vi "Create RPC Method.vi"(8 "error in (no error)":errorcluster, 10 "RPC Method Parameters":T1, 11 "Server class in":refnum<vi>) -> (0 "error out":errorcluster, 2 "Newly created ?":bool, 3 "Server class out":refnum<vi>)   [LabVIEW 2019, in "gRPC Scripting Tools.lvlib"]
uses:
  gRPC Scripting Tools.lvlib
  TypeDefs/RPC Method Parameters.ctl
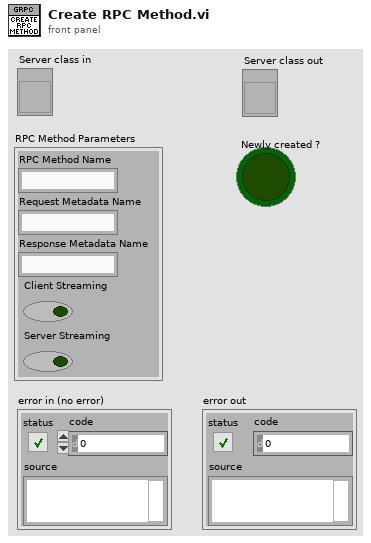
[diagram p1: front panel]
types:
  T1 = typedef "gRPC Scripting Tools.lvlib/RPC Method Parameters.ctl" = cluster{"RPC Method Name":string, "Request Metadata Name":string, "Response Metadata Name":string, "Client Streaming":bool, "Server Streaming":bool}
  T2 = enum32{"invalid VI type", "Standard VI", "Control VI", "Global VI", "Polymorphic VI", "Configuration VI", "SubSystem", "Facade VI", "Method VI"}
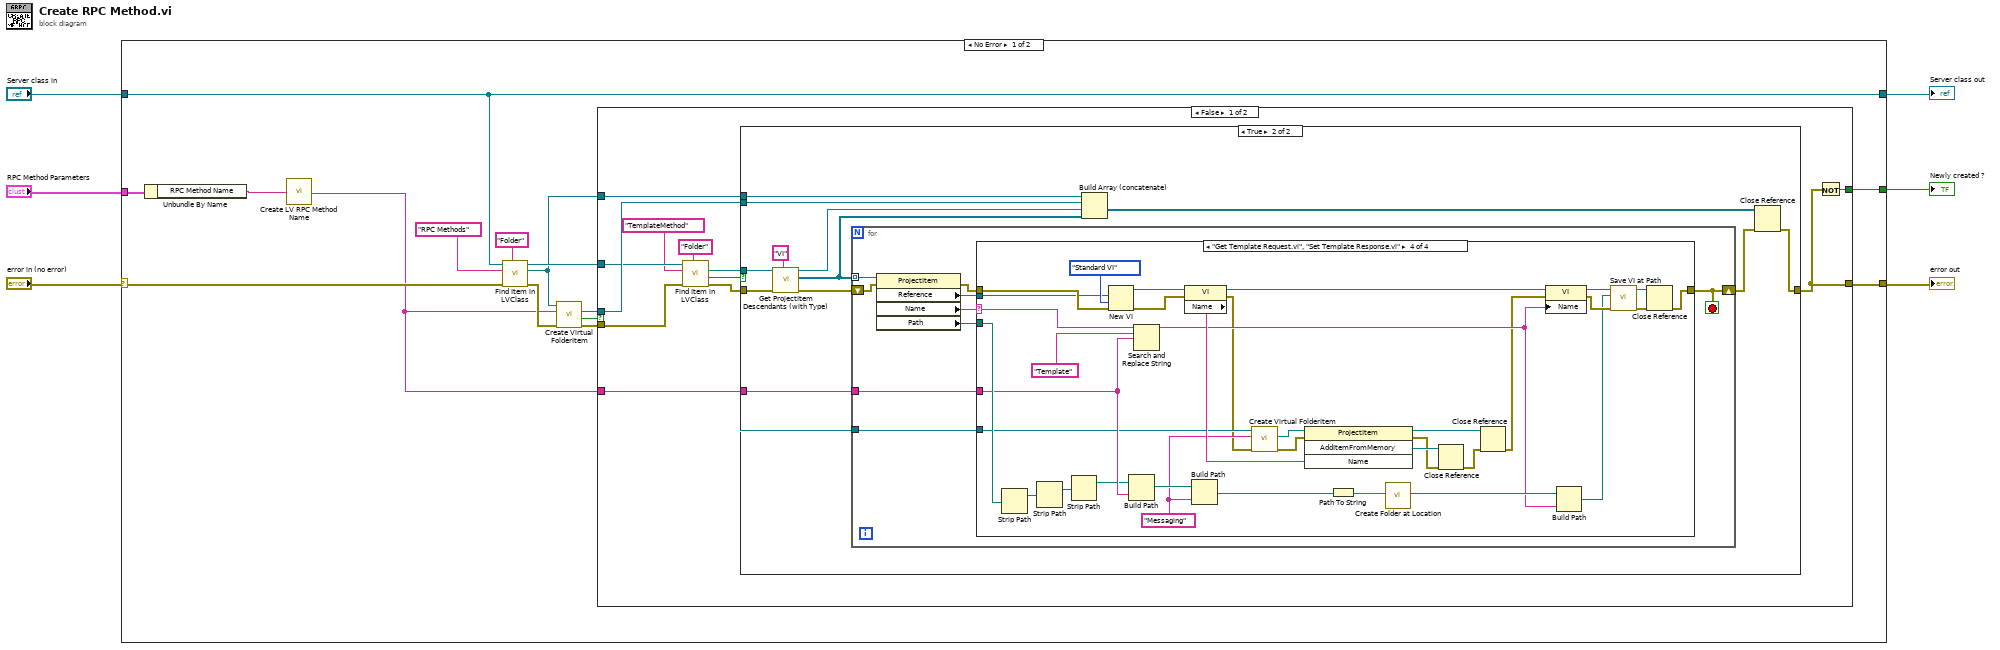
[diagram p0: block diagram]
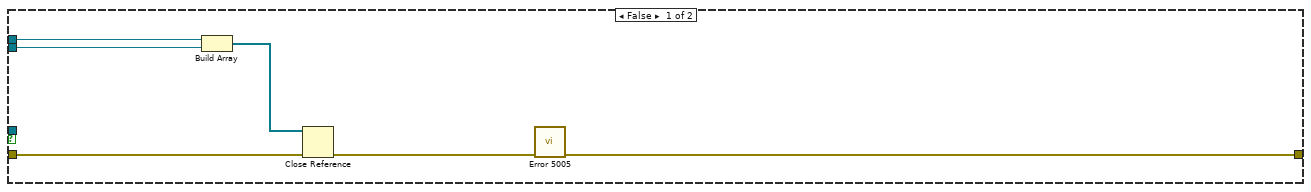
[diagram p2: hidden frame]
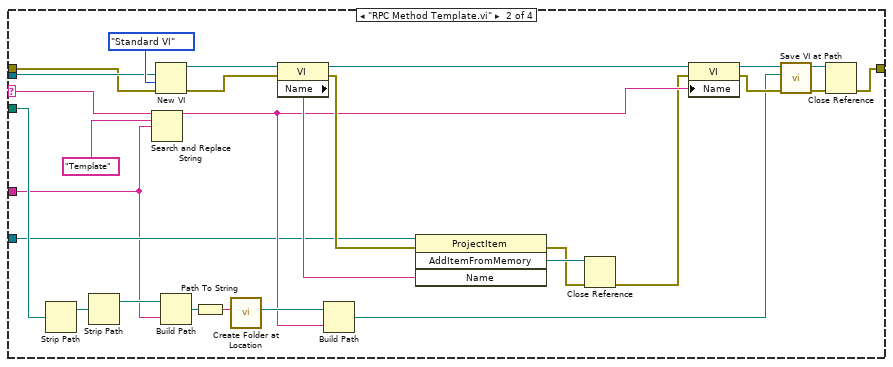
[diagram p4: hidden frame]
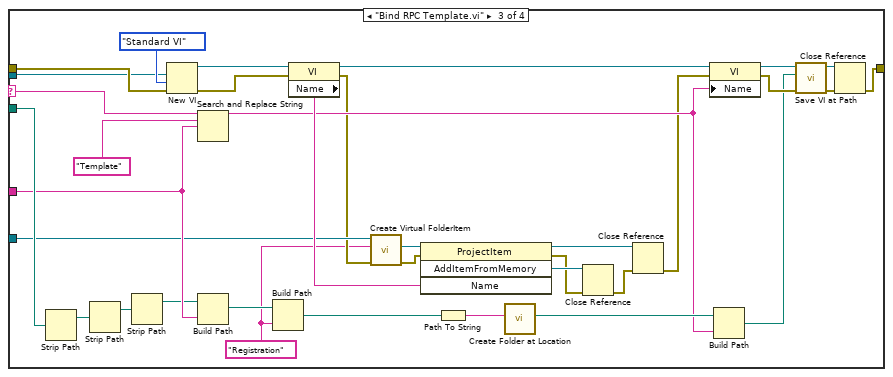
[diagram p5: hidden frame]
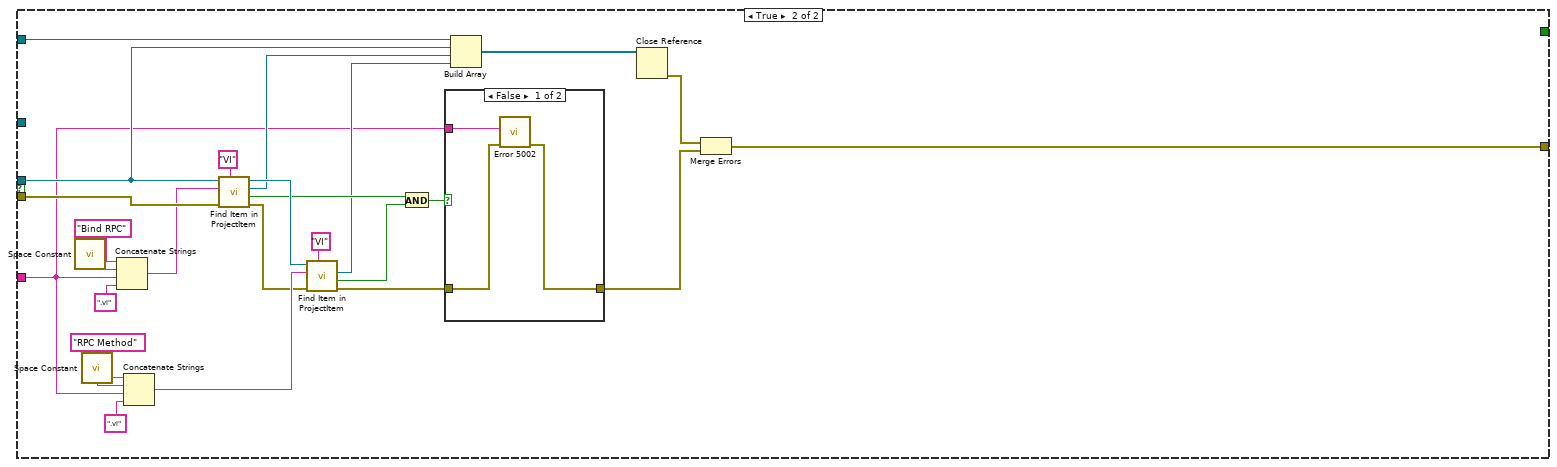
[diagram p6: hidden frame]
diagram:
  n1 = case shown="No Error" "error in (no error)" {
    selector: "error in (no error)" -> [w12 w191]
    tunnel: "Server class in" -> [w11 w190]
    tunnel: [w17 w191] -> w5
    tunnel: [w11 w190] -> w3
    tunnel: [w10 _] -> w2
    tunnel: "RPC Method Parameters" -> [w9 _]
    frame No Error {
      n2 = Unbundle By Name(w9) -> ("RPC Method Name"=w8:string)
      n3 = call "Create LV RPC Method Name.vi"("Proto Parser RPC Method Name in"=w8) -> ("LV RPC Method Name out"=w7:string)
      n4 = call "Find Item in LVClass.vi"("Item Type"="Folder", "error in (no error)"=w12, "Item Name"="RPC Methods", "Class Item in"=w11) -> ("error out"=w16:errorcluster, "Project Item (Class Item)"=w14:refnum<vi>, "Class Item out"=w18:refnum<vi>)  [unwired: 4 in, 1 out]
      n5 = call "Create Virtual FolderItem.vi"("error in (no error)"=w16, "Folder Name"=w7, "ProjectItem in"=w14) -> ("error out"=w15:errorcluster, "Already exists?"=w21:bool, "FolderItem reference out"=w13:refnum<vi>)  [unwired: 5 in, 1 out]
      n6 = case shown="False" w21 {
        tunnel: w13 -> [w33 w168]
        tunnel: w14 -> [w32 w169]
        tunnel: w15 -> [w31 w184]
        tunnel: [w26 w160] -> w17
        tunnel: w18 -> [w30 _]
        tunnel: w7 -> [w27 w164]
        tunnel: [w25 _] -> w10
        frame False {
          n7 = call "Find Item in LVClass.vi"("Item Type"="Folder", "error in (no error)"=w31, "Item Name"="TemplateMethod", "Class Item in"=w30) -> ("error out"=w23:errorcluster, "Found?"=w22:bool, "Project Item (Class Item)"=w24:refnum<vi>)  [unwired: 4 in, 1 out]
          n8 = case shown="True" w22 {
            tunnel: w33 -> [w37 w51]
            tunnel: w32 -> [w38 w50]
            tunnel: w27 -> [_ w48]
            tunnel: [w39 w47] -> w26
            tunnel: w24 -> [_ w46]
            tunnel: w23 -> [w36 w45]
            frame False {
              n9 = Build Array(w38, w37) -> (w35:refnum<vi>[])
              n10 = Close Reference(reference=w35, error in (no error)=w36) -> (error out=w34:errorcluster)
              n11 = call "Error 5005.vi"("error in (no error)"=w34) -> ("error out"=w39:errorcluster)  [unwired: 10 in]
            }
            frame True {
              n12 = call "Get ProjectItem Descendants (with Type).vi"("Type"="VI", "error in (no error)"=w45, "ProjectItem in"=w46) -> ("error out"=w41:errorcluster, "All Descendents"=w42:refnum<vi>[], "ProjectItem out"=w43:refnum<vi>)  [unwired: 6 in]
              n13 = for {
                tunnel: w42 -> [w60] mode=indexing
                tunnel: w51 -> [w54]
                tunnel: w48 -> [w55]
                shift-right: [w52] -> w40
                shift-left: w41 -> [w59]
                stop <- w52 stop-if-true
                n14 = property class="ProjectItem"(reference=w60, error in=w59) -> (error out=w53:errorcluster, "Reference"=w57:refnum<vi>, "Name"=w58:string, "Path"=w56:path)  [unwired: 1 out]
                n15 = case shown="\"Get Template Request.vi\", \"Set Template Response.vi\"" w58 {
                  selector: w58 -> [_ w67 w105 w138]
                  tunnel: w57 -> [_ w68 w106 w139]
                  tunnel: w56 -> [_ w66 w104 w137]
                  tunnel: w55 -> [_ w62 w103 w136]
                  tunnel: w54 -> [_ w65 w97 w132]
                  tunnel: w53 -> [w61 w64 w107 w140]
                  tunnel: [w61 w63 w100 w135] -> w52
                  frame "None", Default {
                  }
                  frame "RPC Method Template.vi" {
                    n16 = Strip Path(path=w66) -> (stripped path=w69:path)  [unwired: 1 out]
                    n17 = Strip Path(path=w69) -> (stripped path=w80:path)  [unwired: 1 out]
                    n18 = Search and Replace String(input string=w67, search string="Template", replace string=w62) -> (result string=w76:string)  [unwired: 5 in, 3 out]
                    n19 = New VI(8:w64, 9:T2."Standard VI" ("vi type (standard vi)"), 10:w68) -> (0:w84:errorcluster, 3:w87:refnum<vi>)  [unwired: 1 in, 3 out]
                    n20 = Build Path(base path=w80, name or relative path=w62) -> (appended path=w79:path)
                    n21 = Path To String(path=w79) -> (string=w78:string)
                    n22 = call "Create Folder at Location.vi"("Path"=w78) -> ("Full path out"=w77:path)  [unwired: 8 in, 2 out]
                    n23 = property class="VI"(reference=w87, error in=w84) -> (reference out=w85:refnum<vi>, error out=w83:errorcluster, "Name"=w88:string)
                    n24 = Build Path(base path=w77, name or relative path=w76) -> (appended path=w75:path)
                    n25 = invoke class="ProjectItem" method="AddItemFromMemory"(reference=w65, error in=w83, "Name"=w88) -> (error out=w71:errorcluster, "AddItemFromMemory"=w72:refnum<vi>)  [unwired: 1 in, 2 out]
                    n26 = Close Reference(reference=w72, error in (no error)=w71) -> (error out=w70:errorcluster)
                    n27 = property class="VI"(reference=w85, error in=w70, "Name"=w76) -> (reference out=w82:refnum<vi>, error out=w81:errorcluster)
                    n28 = call "Save VI at Path.vi"("error in (no error)"=w81, "Path"=w75, "VI in"=w82) -> ("error out"=w74:errorcluster, "VI out"=w73:refnum<vi>)  [unwired: 6 in, 1 out]
                    n29 = Close Reference(reference=w73, error in (no error)=w74) -> (error out=w63:errorcluster)
                  }
                  frame "Bind RPC Template.vi" {
                    w95 = "Registration" ("name or relative path")
                    n30 = Strip Path(path=w104) -> (stripped path=w108:path)  [unwired: 1 out]
                    n31 = Strip Path(path=w108) -> (stripped path=w99:path)  [unwired: 1 out]
                    n32 = Strip Path(path=w99) -> (stripped path=w98:path)  [unwired: 1 out]
                    n33 = New VI(8:w107, 9:T2."Standard VI" ("vi type (standard vi)"), 10:w106) -> (0:w119:errorcluster, 3:w122:refnum<vi>)  [unwired: 1 in, 3 out]
                    n34 = Search and Replace String(input string=w105, search string="Template", replace string=w103) -> (result string=w114:string)  [unwired: 5 in, 3 out]
                    n35 = Build Path(base path=w98, name or relative path=w103) -> (appended path=w102:path)
                    n36 = Build Path(base path=w102, name or relative path=w95) -> (appended path=w101:path)
                    n37 = property class="VI"(reference=w122, error in=w119) -> (reference out=w120:refnum<vi>, error out=w96:errorcluster, "Name"=w123:string)
                    n38 = call "Create Virtual FolderItem.vi"("error in (no error)"=w96, "Folder Name"=w95, "ProjectItem in"=w97) -> ("error out"=w93:errorcluster, "FolderItem reference out"=w94:refnum<vi>)  [unwired: 5 in, 2 out]
                    n39 = invoke class="ProjectItem" method="AddItemFromMemory"(reference=w94, error in=w93, "Name"=w123) -> (reference out=w92:refnum<vi>, error out=w109:errorcluster, "AddItemFromMemory"=w110:refnum<vi>)  [unwired: 1 in, 1 out]
                    n40 = Path To String(path=w101) -> (string=w116:string)
                    n41 = call "Create Folder at Location.vi"("Path"=w116) -> ("Full path out"=w115:path)  [unwired: 8 in, 2 out]
                    n42 = Close Reference(reference=w110, error in (no error)=w109) -> (error out=w91:errorcluster)
                    n43 = Close Reference(reference=w92, error in (no error)=w91) -> (error out=w90:errorcluster)
                    n44 = property class="VI"(reference=w120, error in=w90, "Name"=w114) -> (reference out=w118:refnum<vi>, error out=w117:errorcluster)
                    n45 = Build Path(base path=w115, name or relative path=w114) -> (appended path=w113:path)
                    n46 = call "Save VI at Path.vi"("error in (no error)"=w117, "Path"=w113, "VI in"=w118) -> ("error out"=w112:errorcluster, "VI out"=w111:refnum<vi>)  [unwired: 6 in, 1 out]
                    n47 = Close Reference(reference=w111, error in (no error)=w112) -> (error out=w100:errorcluster)
                  }
                  frame "Get Template Request.vi", "Set Template Response.vi" {
                    w129 = "Messaging" ("name or relative path")
                    n48 = Strip Path(path=w137) -> (stripped path=w143:path)  [unwired: 1 out]
                    n49 = Strip Path(path=w143) -> (stripped path=w134:path)  [unwired: 1 out]
                    n50 = Strip Path(path=w134) -> (stripped path=w133:path)  [unwired: 1 out]
                    n51 = New VI(8:w140, 9:T2."Standard VI" ("vi type (standard vi)"), 10:w139) -> (0:w154:errorcluster, 3:w157:refnum<vi>)  [unwired: 1 in, 3 out]
                    n52 = Build Path(base path=w133, name or relative path=w136) -> (appended path=w142:path)
                    n53 = Search and Replace String(input string=w138, search string="Template", replace string=w136) -> (result string=w149:string)  [unwired: 5 in, 3 out]
                    n54 = property class="VI"(reference=w157, error in=w154) -> (reference out=w155:refnum<vi>, error out=w128:errorcluster, "Name"=w158:string)
                    n55 = Build Path(base path=w142, name or relative path=w129) -> (appended path=w141:path)
                    n56 = call "Create Virtual FolderItem.vi"("error in (no error)"=w128, "Folder Name"=w129, "ProjectItem in"=w132) -> ("error out"=w130:errorcluster, "FolderItem reference out"=w131:refnum<vi>)  [unwired: 5 in, 2 out]
                    n57 = invoke class="ProjectItem" method="AddItemFromMemory"(reference=w131, error in=w130, "Name"=w158) -> (reference out=w127:refnum<vi>, error out=w144:errorcluster, "AddItemFromMemory"=w145:refnum<vi>)  [unwired: 1 in, 1 out]
                    n58 = Path To String(path=w141) -> (string=w151:string)
                    n59 = call "Create Folder at Location.vi"("Path"=w151) -> ("Full path out"=w150:path)  [unwired: 8 in, 2 out]
                    n60 = Close Reference(reference=w145, error in (no error)=w144) -> (error out=w126:errorcluster)
                    n61 = Close Reference(reference=w127, error in (no error)=w126) -> (error out=w125:errorcluster)
                    n62 = property class="VI"(reference=w155, error in=w125, "Name"=w149) -> (reference out=w153:refnum<vi>, error out=w152:errorcluster)
                    n63 = Build Path(base path=w150, name or relative path=w149) -> (appended path=w148:path)
                    n64 = call "Save VI at Path.vi"("error in (no error)"=w152, "Path"=w148, "VI in"=w153) -> ("error out"=w147:errorcluster, "VI out"=w146:refnum<vi>)  [unwired: 6 in, 1 out]
                    n65 = Close Reference(reference=w146, error in (no error)=w147) -> (error out=w135:errorcluster)
                  }
                }
              }
              n66 = Build Array (concatenate)(w50, w51, w43, w42) -> (w49:refnum<vi>[])
              n67 = Close Reference(reference=w49, error in (no error)=w40) -> (error out=w47:errorcluster)
            }
          }
          n68 = Not(x=w26) -> (.not. x?=w25:bool)
        }
        frame True {
          n69 = call <vilib>:"Space Constant.vi"() -> ("String"=w177:string)
          n70 = call <vilib>:"Space Constant.vi"() -> ("String"=w176:string)
          n71 = Concatenate Strings("Bind RPC" ("string"), w177, w164, ".vi" ("string")) -> (w180:string)
          n72 = Concatenate Strings("RPC Method" ("string"), w176, w164, ".vi" ("string")) -> (w174:string)
          n73 = call "Find Item in ProjectItem.vi"("Item Type"="VI" ("Type"), "error in (no error)"=w184, "Name"=w180, "ProjectItem in"=w168) -> ("error out"=w173:errorcluster, "Found ?"=w172:bool, "Item Refnum out"=w167:refnum<vi>, "ProjectItem out"=w182:refnum<vi>)  [unwired: 4 in]
          n74 = call "Find Item in ProjectItem.vi"("Item Type"="VI" ("Type"), "error in (no error)"=w173, "Name"=w174, "ProjectItem in"=w182) -> ("error out"=w165:errorcluster, "Found ?"=w171:bool, "Item Refnum out"=w166:refnum<vi>)  [unwired: 4 in, 1 out]
          n75 = And(x=w172, y=w171) -> (x .and. y?=w170:bool)
          n76 = case shown="False" w170 {
            tunnel: w165 -> [w188 w189]
            tunnel: w164 -> [w186 _]
            tunnel: [w187 w189] -> w162
            frame False {
              n77 = call "Error 5002.vi"("error in (no error)"=w188, "Method Name"=w186) -> ("error out"=w187:errorcluster)  [unwired: 9 in]
            }
            frame True {
            }
          }
          n78 = Build Array(w169, w168, w167, w166) -> (w163:refnum<vi>[])
          n79 = Close Reference(reference=w163) -> (error out=w161:errorcluster)  [unwired: 1 in]
          n80 = Merge Errors(w161, w162) -> (w160:errorcluster)
        }
      }
    }
    frame Error {
    }
  }
  "error out" <- w5
  "Server class out" <- w3
  "Newly created ?" <- w2
